vi "SQUARED_JOYSTICK.vi"(11 "axis input":dbl) -> (3 "axis output":dbl)   [LabVIEW 2014]
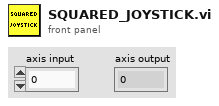
[diagram p1: front panel]
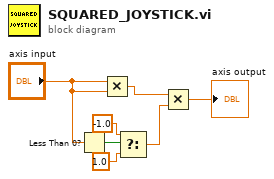
[diagram p0: block diagram]
diagram:
  n1 = Less Than 0?(x="axis input") -> (x < 0?=w4:bool)
  n2 = Multiply(x="axis input", y="axis input") -> (x*y=w6:dbl)
  n3 = Select(t=-1.0, s=w4, f=1.0) -> (s? t:f=w1:dbl)
  n4 = Multiply(x=w6, y=w1) -> (x*y=→"axis output":dbl)
